vi "SwerveDriveFuse.vi"(0 "Strafe Joystick Axes":cluster{"X":dbl, "Y":dbl}, 1 "Face Joystick Axes":cluster{"X":dbl, "Y":dbl}, 2 "Trigger Axes/Turn Speed":cluster{"Left":dbl, "Right":dbl}, 3 "Face PID Gains":T1={"proportional gain (Kc)"=0.275, "integral time (Ti, min)"=0.0, "derivative time (Td, min)"=0.006} {"derivative time (Td, min)" format="%.3f"; "integral time (Ti, min)" format="%.3f"; "proportional gain (Kc)" format="%.3f"}, 4 "Angle (degrees; 0 = right)":dbl, 5 "error in (no error)":errorcluster, 6 "Strafe Multiplier":dbl, 8 "Rotation Multiplier":dbl, 10 "Max Wheel Speed":dbl) -> (16 "Speed Chart":cluster{dbl, "Encoder Velocity":dbl}[](graph), 19 "error out":errorcluster)   [LabVIEW 2015]
uses:
  Team900SwerveDrive.lvlib
  SwerveDriveFace.vi
  SwerveDriveRotate.vi
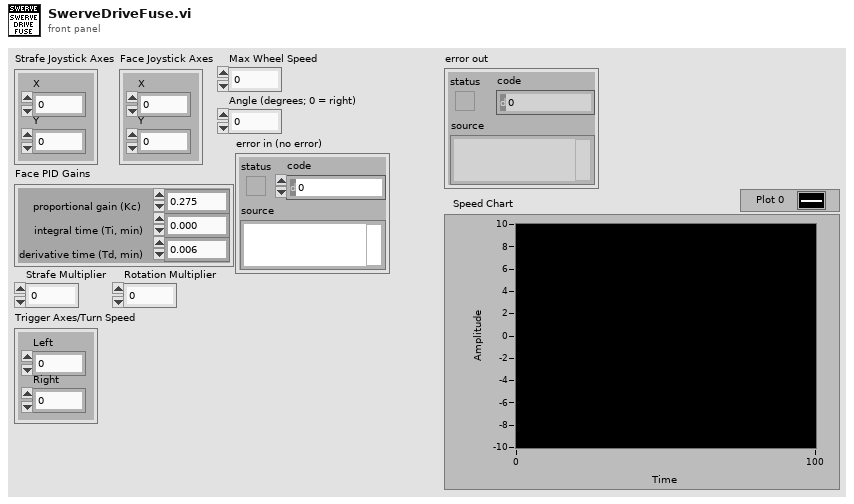
[diagram p1: front panel]
types:
  T1 = cluster{"proportional gain (Kc)":dbl, "integral time (Ti, min)":dbl, "derivative time (Td, min)":dbl}
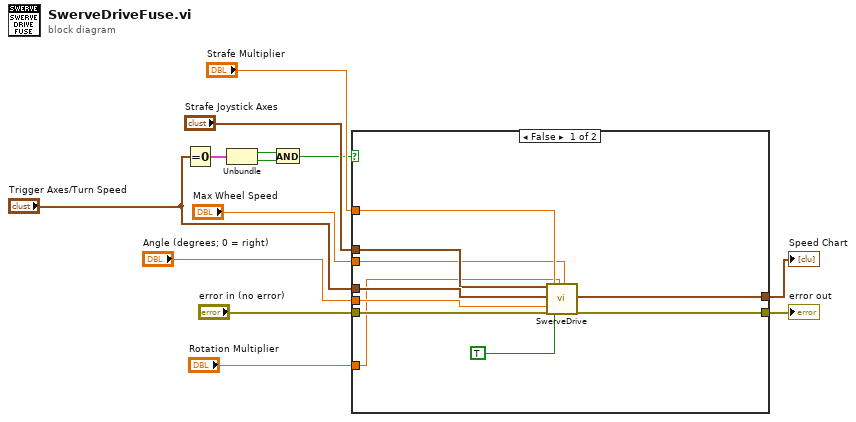
[diagram p0: block diagram]
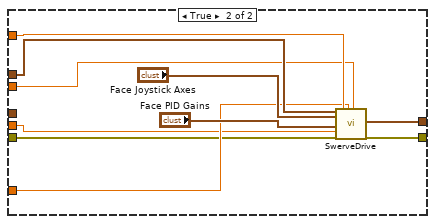
[diagram p2: hidden frame]
diagram:
  n1 = Equal To 0?(x="Trigger Axes/Turn Speed") -> (x = 0?=w6:cluster{"Left":bool, "Right":bool})
  n2 = Unbundle(w6) -> ("Left"=w5:bool, "Right"=w4:bool)
  n3 = And(x=w5, y=w4) -> (x .and. y?=w3:bool)
  n4 = case shown="False" w3 {
    tunnel: "Strafe Joystick Axes" -> [w19 w33]
    tunnel: "Strafe Multiplier" -> [w17 w30]
    tunnel: "Rotation Multiplier" -> [w16 w29]
    tunnel: "Max Wheel Speed" -> [w15 w28]
    tunnel: "Angle (degrees; 0 = right)" -> [w18 w27]
    tunnel: "error in (no error)" -> [w22 w26]
    tunnel: [w23 w25] -> w7
    tunnel: "Trigger Axes/Turn Speed" -> [w20 _]
    tunnel: [w14 w24] -> w1
    frame False {
      n5 = call-poly "SwerveDrive.vi"("Strafe Joystick Axes"=w19, "Trigger Axes"=w20, "Angle (degrees; 0 = right)"=w18, "error in (no error)"=w22, "Strafe Multiplier"=w17, "FieldCentric? (T)"=TRUE, "Rotation Multiplier"=w16, "Max Wheel Speed"=w15) -> ("Speed Chart"=w14:cluster{dbl, "Encoder Velocity":dbl}[], "error out"=w23:errorcluster)  [unwired: 9 in, 1 out]
    }
    frame True {
      n6 = call-poly "SwerveDrive.vi"("Strafe Joystick Axes"=w33, "Face Joystick Axes"="Face Joystick Axes", "Face PID Gains"="Face PID Gains", "Angle (degrees; 0 = right)"=w27, "error in (no error)"=w26, "Strafe Multiplier"=w30, "Rotation Multiplier"=w29, "Max Wheel Speed"=w28) -> ("Speed Chart"=w24:cluster{dbl, "Encoder Velocity":dbl}[], "error out"=w25:errorcluster)  [unwired: 10 in]
    }
  }
  "error out" <- w7
  "Speed Chart" <- w1
